vi "command interface.vi"(7 "Max time (ms) (2000)":u32=2000, 8 "Parameter":string, 9 "command":string, 10 "Serial Port":refnum<visa-resource-name>) -> (0 "timed out":bool, 1 "return code":string, 2 "response":string="3", 3 "Serial Port":refnum<visa-resource-name>)   [LabVIEW 2012]
doc: "The default termination sequence is \"return\".\nThe default command introducer is \"escC\"."
panel:
  in  "description":string[](array[string])=["Enable even parity", "Enable odd parity", "disable parity [default]", "Set HP 5890 default configuration", "Enable echo", "Disable echo [default]", "Enable host handshake -ENQ/ACK", "Disable host handshake [default]", "Enable HP 5890 (node) handshake -ENQ/ACK [default]", "Disable HP 5890 (node) handshake", "Define read sequence [default (none)]", "Define termination sequence [default (CR/LF)]", "Enable XON/XOFF protocol", "Disable XON/XOFF protocol [default]", "Acquire or release remote control; locks keyboard", "read actual temperatures and flows", "Change all; send a workfile to HP 5890", "Read HP 5890 environmental status", "read HP 5890 instrument configuration", "read HP 5890 instrument fault string", "read last HP 5890 key pressed", "List all; receive a workfile from HP 5890", "lock or unlock the start key", "ouput text to the HP 5890 display", "read HP 5890 serial interface fault word", "read run and readiness information", "perform remote keystrokes from the host", "retransmit last message sent by the HP 5890", "delays start until host is ready", "requests that the host be notified when HP 5890 status is modified", "start notification when HP 5890 begins to run", "configure data transfer", "configure signal producers", "send signal data"]
  in  "command code":string[](array[string])=["EP", "OP", "ZP", "DF", "E+", "E-", "H+", "H-", "N+", "N-", "RS", "TS", "X+", "X-", "AR", "AT", "CA", "EV", "IC", "IF", "IK", "LA", "LU", "OT", "RF", "RI", "RK", "RT", "HR", "SM", "ST", "CD", "CP", "SD"]
  in  "End":string
  in  "Commence":string
  in  "abort":string
  in  "termination sequence":string="\n"
  in  "command introducer":string="\u001bC"
  in  "stages":T1(array[ring])=[enum."1 stage", enum."1 stage", enum."1 stage", enum."1 stage", enum."1 stage", enum."1 stage", enum."1 stage", enum."1 stage", enum."1 stage", enum."1 stage", enum."1 stage", enum."1 stage", enum."1 stage", enum."1 stage", enum."4 stage", enum."2 stage", enum."change all", enum."2 stage", enum."2 stage", enum."2 stage", enum."2 stage", enum."list all", enum."4 stage", enum."4 stage", enum."2 stage", enum."2 stage", enum."4 stage", enum."2 stage", enum."2 stage", enum."3 stage", enum."2 stage", enum."4 stage", enum."4 stage", enum."data stream"]
  # "First you need to run Serial init vi,  then TS with #/n# as parameter in this VI."
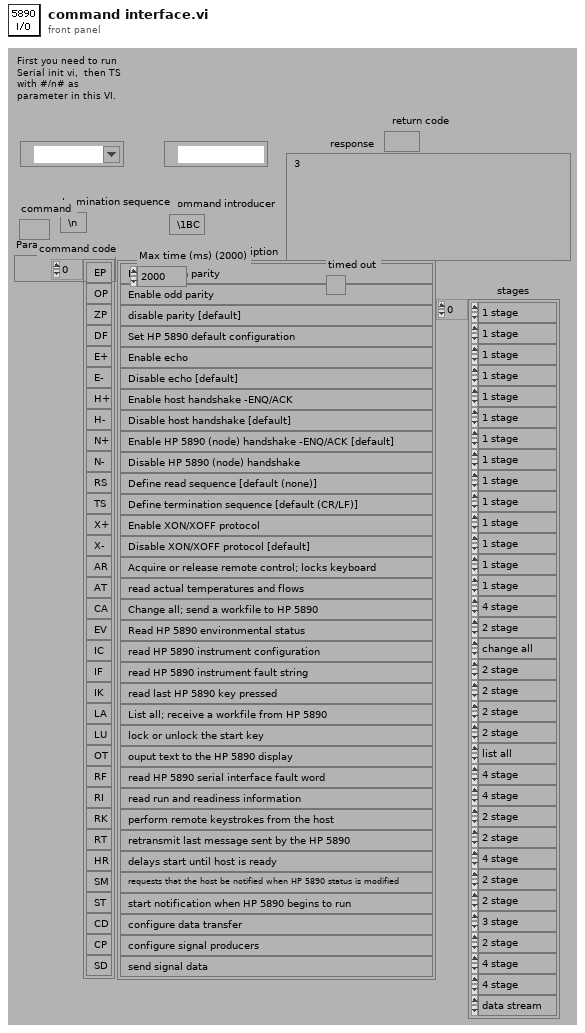
[diagram p1: front panel]
types:
  T1 = enum16{"1 stage", "2 stage", "3 stage", "4 stage", "change all", "list all", "data stream"}[]
  T2 = enum16{"1 stage", "2 stage", "3 stage", "4 stage", "change all", "list all", "data stream"}
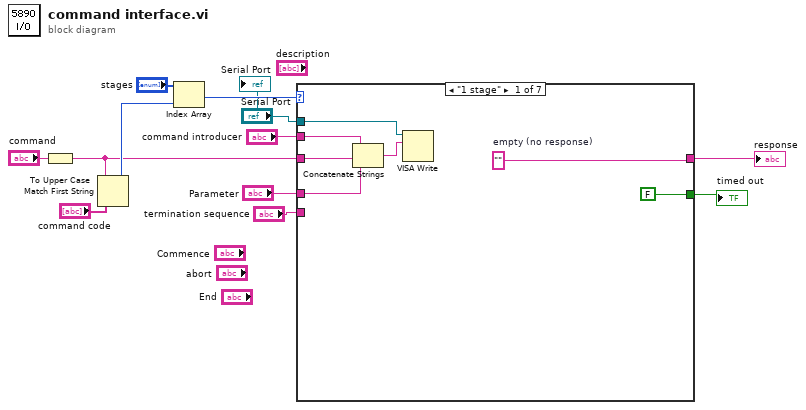
[diagram p0: block diagram]
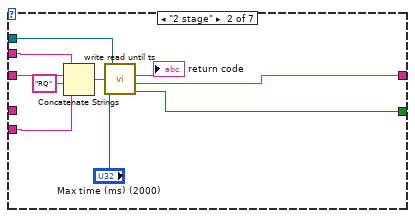
[diagram p2: hidden frame]
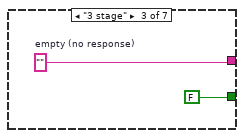
[diagram p3: hidden frame]
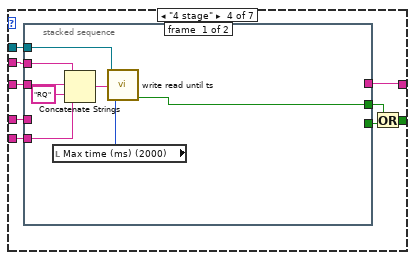
[diagram p4: hidden frame]
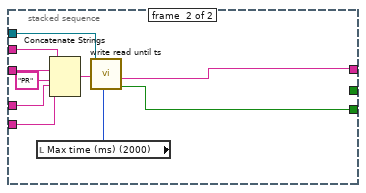
[diagram p5: hidden frame]
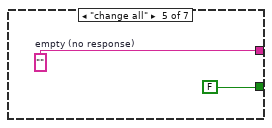
[diagram p6: hidden frame]
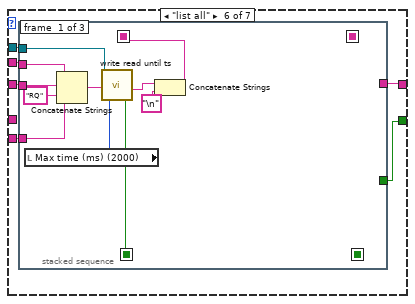
[diagram p7: hidden frame]
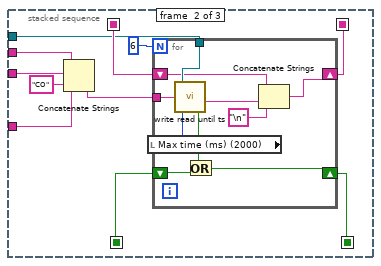
[diagram p8: hidden frame]
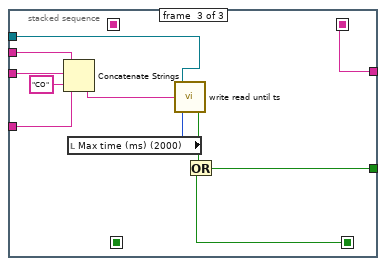
[diagram p9: hidden frame]
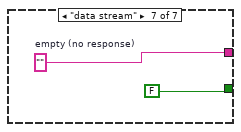
[diagram p10: hidden frame]
diagram:
  n1 = To Upper Case(1:"command") -> (0:w3:string)
  n2 = Match First String(2:"command code", 3:w3) -> (0:w5:i32)  [unwired: 1 out]
  n3 = Index Array(array="stages", index=w5) -> (element=w4:T2)
  n4 = case shown="\"1 stage\"" w4 {
    tunnel: "Serial Port" -> [w14 w26 _ w40 _ w66 _]
    tunnel: "command introducer" -> [w19 w29 _ w39 _ w65 _]
    tunnel: w3 -> [w18 w28 _ w37 _ w64 _]
    tunnel: "termination sequence" -> [_ w25 _ w38 _ w63 _]
    tunnel: [w17 w24 w31 w35 w60 w62 w111] -> w10
    tunnel: "Parameter" -> [w16 _ _ w36 _ _ _]
    tunnel: [FALSE w20 FALSE w33 FALSE w61 FALSE] -> w2
    frame "1 stage" {
      w17 = ""  # empty (no response)
      n5 = Concatenate Strings(w19, w18, w16) -> (w13:string)
      n6 = VISA Write(VISA resource name=w14, write buffer=w13) -> ()  [unwired: 1 in, 3 out]
    }
    frame "2 stage" {
      n7 = Concatenate Strings(w29, w28, "RQ", w25) -> (w23:string)
      n8 = call "write read until ts.vi"("Max time (ms) (2000)"="Max time (ms) (2000)", "string to write"=w23, "Port Number"=w26) -> ("Time out"=w20:bool, "return string"=w24:string, "return code"=→"return code":string)  [unwired: 1 in, 1 out]
    }
    frame "3 stage" {
      w31 = ""  # empty (no response)
    }
    frame "4 stage" {
      n9 = stacked-sequence {
        tunnel: w37 -> [w47 w57]
        tunnel: w38 -> [w43 w53]
        tunnel: w39 -> [w45 w56]
        tunnel: w40 -> [w44 w54]
        tunnel: w36 -> [_ w55]
        tunnel: [_ w52] -> w35
        tunnel: [_ w49] -> w34
        tunnel: [w41 _] -> w32
        frame #0 {
          n10 = local read "Max time (ms) (2000)"() -> (w42:u32)
          n11 = Concatenate Strings(w45, w47, "RQ", w43) -> (w46:string)
          n12 = call "write read until ts.vi"("Max time (ms) (2000)"=w42, "string to write"=w46, "Port Number"=w44) -> ("Time out"=w41:bool)  [unwired: 1 in, 3 out]
        }
        frame #1 {
          n13 = local read "Max time (ms) (2000)"() -> (w50:u32)
          n14 = Concatenate Strings(w56, w57, "PR", w55, w53) -> (w51:string)
          n15 = call "write read until ts.vi"("Max time (ms) (2000)"=w50, "string to write"=w51, "Port Number"=w54) -> ("Time out"=w49:bool, "return string"=w52:string)  [unwired: 1 in, 2 out]
        }
      }
      n16 = Or(x=w32, y=w34) -> (x .or. y?=w33:bool)
    }
    frame "change all" {
      w60 = ""  # empty (no response)
    }
    frame "list all" {
      n17 = stacked-sequence {
        seq-local: [w68 _ _] -> [_ w83 _]
        seq-local: [w71 _ _] -> [_ w80 _]
        seq-local: [_ w79 _] -> [_ _ w102]
        seq-local: [_ w78 _] -> [_ _ w101]
        tunnel: w63 -> [w72 w88 w109]
        tunnel: w64 -> [w77 w87 w108]
        tunnel: w65 -> [w76 w86 w107]
        tunnel: w66 -> [w73 w81 w104]
        tunnel: [_ _ w102] -> w62
        tunnel: [_ _ w99] -> w61
        frame #0 {
          n18 = local read "Max time (ms) (2000)"() -> (w69:u32)
          n19 = Concatenate Strings(w76, w77, "RQ", w72) -> (w75:string)
          n20 = call "write read until ts.vi"("Max time (ms) (2000)"=w69, "string to write"=w75, "Port Number"=w73) -> ("Time out"=w71:bool, "return string"=w70:string)  [unwired: 1 in, 2 out]
          n21 = Concatenate Strings(w70, "\n") -> (w68:string)
        }
        frame #1 {
          n22 = Concatenate Strings(w86, w87, "CO", w88) -> (w82:string)
          n23 = for {
            N: 6 -> [_]
            shift-right: [w95] -> w79
            shift-left: w83 -> [w96]
            tunnel: w82 -> [w94]
            tunnel: w81 -> [w98]
            shift-right: [w91] -> w78
            shift-left: w80 -> [w92]
            n24 = local read "Max time (ms) (2000)"() -> (w89:u32)
            n25 = call "write read until ts.vi"("Max time (ms) (2000)"=w89, "string to write"=w94, "Port Number"=w98) -> ("Time out"=w93:bool, "return string"=w97:string)  [unwired: 1 in, 2 out]
            n26 = Or(x=w93, y=w92) -> (x .or. y?=w91:bool)
            n27 = Concatenate Strings(w96, w97, "\n") -> (w95:string)
          }
        }
        frame #2 {
          n28 = Concatenate Strings(w107, w108, "CO", w109) -> (w105:string)
          n29 = local read "Max time (ms) (2000)"() -> (w100:u32)
          n30 = call "write read until ts.vi"("Max time (ms) (2000)"=w100, "string to write"=w105, "Port Number"=w104) -> ("Time out"=w103:bool)  [unwired: 1 in, 3 out]
          n31 = Or(x=w103, y=w101) -> (x .or. y?=w99:bool)
        }
      }
    }
    frame "data stream" {
      w111 = ""  # empty (no response)
    }
  }
  "response" <- w10
  "timed out" <- w2
  "Serial Port" <- "Serial Port"
